vi "write_IFD.vi"(8 "error in":errorcluster, 9 "byte order (0:big-endian, network order)":T2(ring), 10 "Cluster":T3, 11 "tiff_file_input":refnum<file>) -> (0 "error out":errorcluster, 1 "next_IFD_offset_offset":u32, 2 "frame_data_offset":u32, 3 "tiff_file_out":refnum<file>)   [LabVIEW 2013]
doc: "write image file directionary to a tiff file."
panel:
  out "IFD":T1
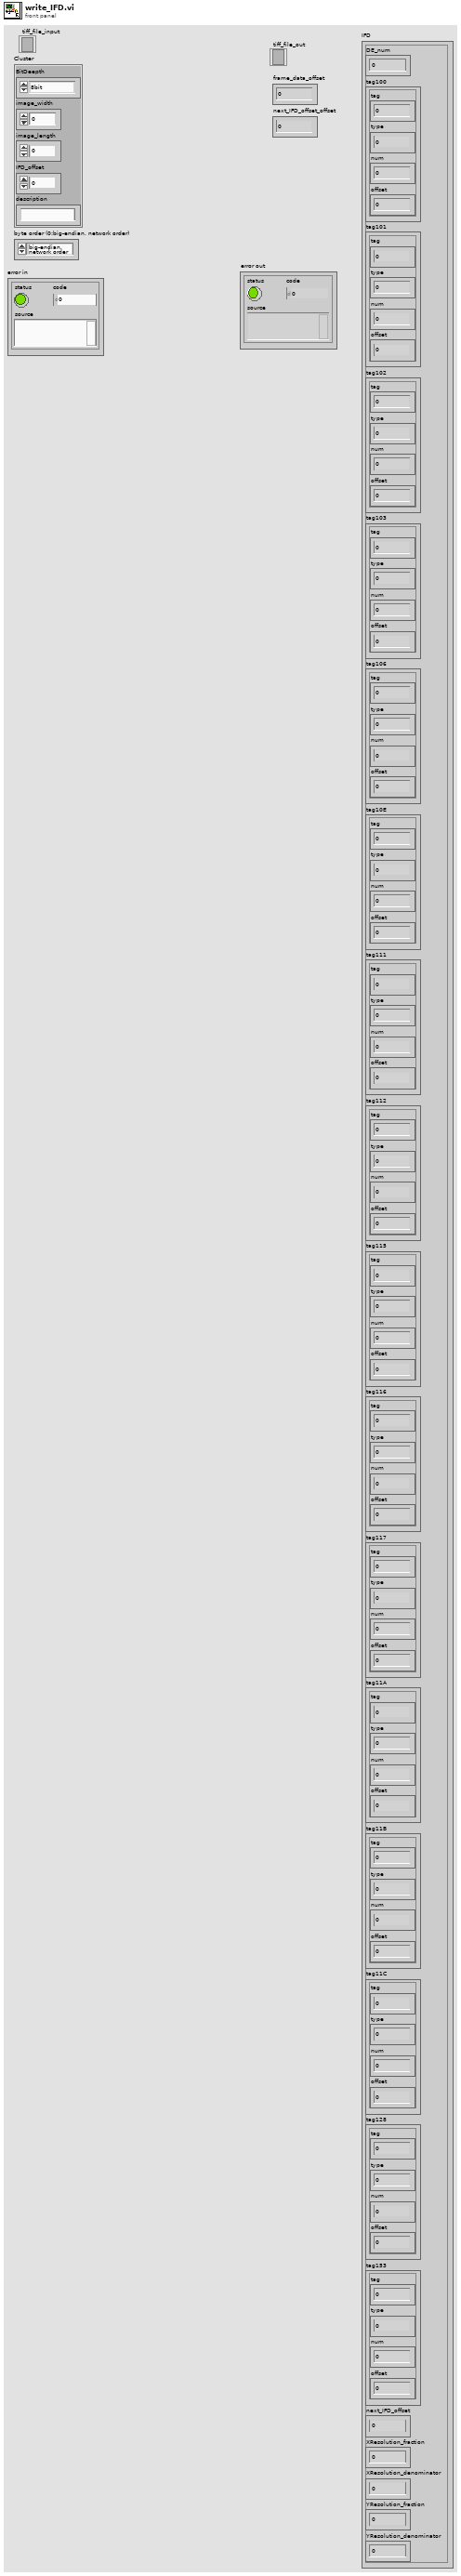
[diagram p1: front panel]
types:
  T1 = cluster{"DE_num":u16, "tag100":cluster{"tag":u16, "type":u16, "num":u32, "offset":u32}, "tag101":cluster{"tag":u16, "type":u16, "num":u32, "offset":u32}, "tag102":cluster{"tag":u16, "type":u16, "num":u32, "offset":u32}, "tag103":cluster{"tag":u16, "type":u16, "num":u32, "offset":u32}, "tag106":cluster{"tag":u16, "type":u16, "num":u32, "offset":u32}, "tag10E":cluster{"tag":u16, "type":u16, "num":u32, "offset":u32}, "tag111":cluster{"tag":u16, "type":u16, "num":u32, "offset":u32}, "tag112":cluster{"tag":u16, "type":u16, "num":u32, "offset":u32}, "tag115":cluster{"tag":u16, "type":u16, "num":u32, "offset":u32}, "tag116":cluster{"tag":u16, "type":u16, "num":u32, "offset":u32}, "tag117":cluster{"tag":u16, "type":u16, "num":u32, "offset":u32}, "tag11A":cluster{"tag":u16, "type":u16, "num":u32, "offset":u32}, "tag11B":cluster{"tag":u16, "type":u16, "num":u32, "offset":u32}, "tag11C":cluster{"tag":u16, "type":u16, "num":u32, "offset":u32}, "tag128":cluster{"tag":u16, "type":u16, "num":u32, "offset":u32}, "tag153":cluster{"tag":u16, "type":u16, "num":u32, "offset":u32}, "next_IFD_offset":u32, "XResolution_fraction":u32, "XResolution_denominator":u32, "YResolution_fraction":u32, "YResolution_denominator":u32}
  T2 = enum16{"big-endian, network order", "native, host order", "little-endian"}
  T3 = cluster{"BitDeepth":enum16{"8bit", "16bit", "32bit"}, "image_width":u32, "image_length":u32, "IFD_offset":u32, "description":string}
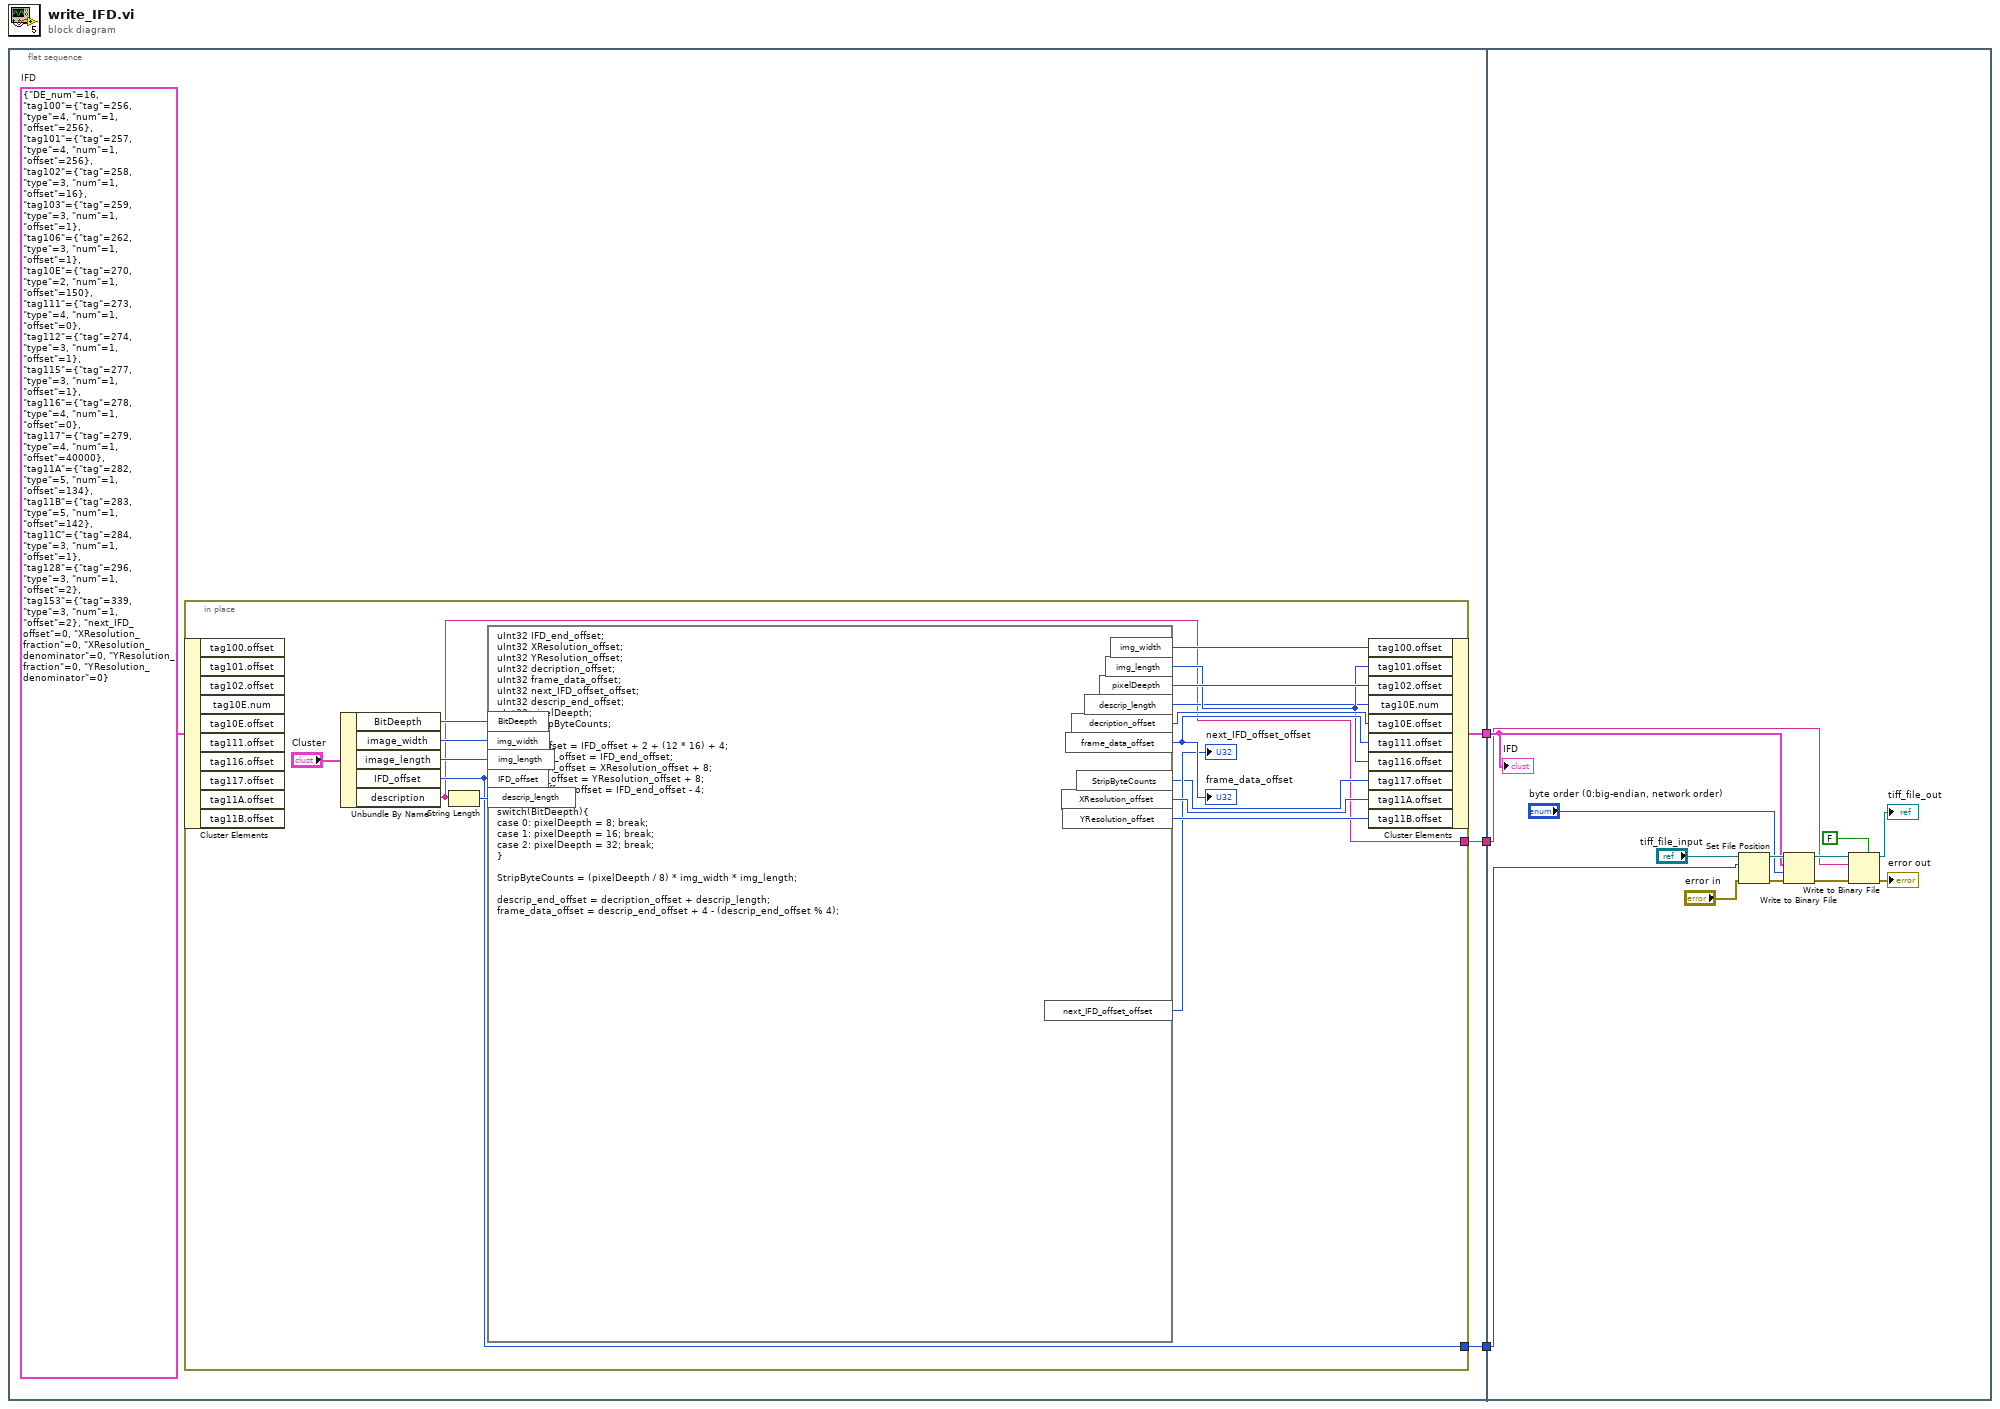
[diagram p0: block diagram]
diagram:
  n1 = flat-sequence {
    tunnel: [w6] -> w3
    tunnel: [w5] -> w2
    tunnel: [w4] -> w1
    tunnel: w3 -> [w31]
    tunnel: w2 -> [w32]
    tunnel: w1 -> [w26]
    frame #0 {
      w7 = T1 {"DE_num"=16, "tag100"={"tag"=256, "type"=4, "num"=1, "offset"=256}, "tag101"={"tag"=257, "type"=4, "num"=1, "offset"=256}, "tag102"={"tag"=258, "type"=3, "num"=1, "offset"=16}, "tag103"={"tag"=259, "type"=3, "num"=1, "offset"=1}, "tag106"={"tag"=262, "type"=3, "num"=1, "offset"=1}, "tag10E"={"tag"=270, "type"=2, "num"=1, "offset"=150}, "tag111"={"tag"=273, "type"=4, "num"=1, "offset"=0}, "tag112"={"tag"=274, "type"=3, "num"=1, "offset"=1}, "tag115"={"tag"=277, "type"=3, "num"=1, "offset"=1}, "tag116"={"tag"=278, "type"=4, "num"=1, "offset"=0}, "tag117"={"tag"=279, "type"=4, "num"=1, "offset"=40000}, "tag11A"={"tag"=282, "type"=5, "num"=1, "offset"=134}, "tag11B"={"tag"=283, "type"=5, "num"=1, "offset"=142}, "tag11C"={"tag"=284, "type"=3, "num"=1, "offset"=1}, "tag128"={"tag"=296, "type"=3, "num"=1, "offset"=2}, "tag153"={"tag"=339, "type"=3, "num"=1, "offset"=2}, "next_IFD_offset"=0, "XResolution_fraction"=0, "XResolution_denominator"=0, "YResolution_fraction"=0, "YResolution_denominator"=0}  # IFD
      n2 = in-place {
        in-place-border: [w9] -> w5
        in-place-border: [w8] -> w4
        n3 = in-place-cluster #1(w7) -> ()  [unwired: 10 out]
        n4 = Unbundle By Name("Cluster") -> ("BitDeepth"=w15:enum16{"8bit", "16bit", "32bit"}, "image_width"=w17:u32, "image_length"=w16:u32, "IFD_offset"=w9:u32, "description"=w8:string)
        n5 = String Length(string=w8) -> (length=w24:i32)
        n6 = formula code="uInt32 IFD_end_offset;\nuInt32 XResolution_offset;\nuInt32 YResolution_offset;\nuInt32 decription_offset;\nuInt32 frame_data_offset;\nuInt32 next_IFD_offset_offset;\nuInt32 descrip_end_offset;\nuInt32 pixelDeepth;\nuInt32 StripByteCounts;\n\nIFD_end_offset = IFD_offset + 2 + (12 * 16) + 4;\nXResolution_offset = IFD_end_offset;\nYResolution_offset = XResolution_offset + 8;\ndecription_offset = YResolution_offset + 8;\nnext_IFD_offset_offset = IFD_end_offset - 4;\n\nswitch(BitDeepth){\ncase 0: pixelDeepth = 8; break;\ncase 1: pixelDeepth = 16; break;\ncase 2: pixelDeepth = 32; break;\n}\n\nStripByteCounts = (pixelDeepth / 8) * img_width * img_length;\n\ndescrip_end_offset = decription_offset + descrip_length;\nframe_data_offset = descrip_end_offset + 4 - (descrip_end_offset % 4);"("IFD_offset"=w9, "descrip_length"=w24, "img_width"=w17, "img_length"=w16, "BitDeepth"=w15) -> ("XResolution_offset"=w21:u32, "YResolution_offset"=w20:u32, "decription_offset"=w23:u32, "frame_data_offset"=w22:u32, "next_IFD_offset_offset"=→"next_IFD_offset_offset":u32, "StripByteCounts"=w14:u32, "pixelDeepth"=w13:u32, "img_length"=w11:u32, "img_width"=w12:u32, "descrip_length"=w10:i32)
        "frame_data_offset" <- w22
        n7 = in-place-cluster #1("tag100.offset"=w12, "tag101.offset"=w11, "tag102.offset"=w13, "tag10E.num"=w10, "tag10E.offset"=w23, "tag111.offset"=w22, "tag116.offset"=w11, "tag117.offset"=w14, "tag11A.offset"=w21, "tag11B.offset"=w20) -> (w6:T1)
      }
    }
    frame #1 {
      n8 = Set File Position(offset (in bytes) (0)=w32, refnum="tiff_file_input", error in="error in") -> (refnum out=w35:refnum<file>, error out=w36:errorcluster)  [unwired: 1 in]
      n9 = Write to Binary File(file (use dialog)=w35, data=w31, error in=w36, 9:"byte order (0:big-endian, network order)") -> (refnum out=w30:refnum<file>, error out=w29:errorcluster)  [unwired: 2 in, 1 out]
      n10 = Write to Binary File(file (use dialog)=w30, data=w26, error in=w29, 5:FALSE ("prepend array or string size? (T)")) -> (refnum out=→"tiff_file_out":refnum<file>, error out=→"error out":errorcluster)  [unwired: 2 in, 1 out]
      "IFD" <- w31
    }
  }
